vi "CreateChanGrp.vi"(8 "error in (no error)":errorcluster, 9 "GroupChans":refnum<class "Channel.lvclass">[](array[class]), 10 "MeasType":T1, 11 "GroupName":string) -> (0 "error out":errorcluster, 3 "ChanGrp out":refnum<class "ChanGrp.lvclass">)   [LabVIEW 2018, in "Configuration Grandmaster.lvlib" / "ChanGrp.lvclass"]
uses:
  ChanGrp.lvclass
  Custom Ctrls/ge_MeasType.ctl
  Measurements/Class Channel/Channel.lvclass
  ChanGrp.lvclass/ChanGrp.ctl
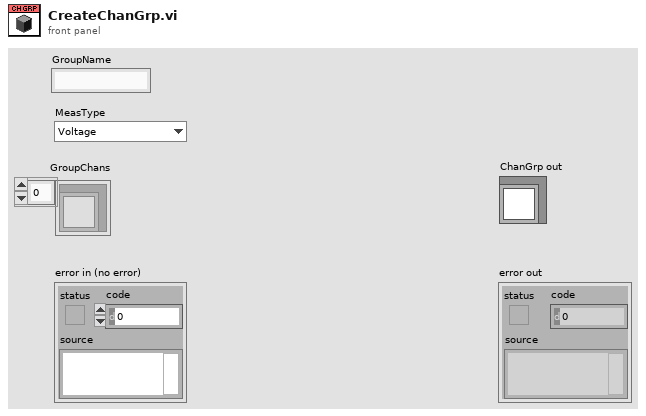
[diagram p1: front panel]
types:
  T1 = typedef "ge_MeasType.ctl" = enum16{"Voltage", "Frequency", "Tachometer", "Dynamic", "Thermocouple", "RTD", "Strain", "Current", "Resistance"}
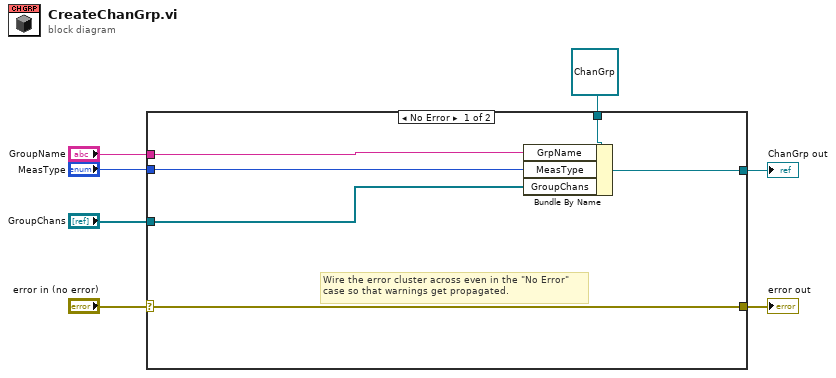
[diagram p0: block diagram]
diagram:
  n1 = case shown="No Error" "error in (no error)" {
    selector: "error in (no error)" -> [w13 w15]
    tunnel: [w13 w15] -> w6
    tunnel: [w11 w14] -> w5
    tunnel: refnum<class "ChanGrp.lvclass"> refnum ("ChanGrp.lvclass") -> [w12 w14]
    tunnel: "GroupName" -> [w10 _]
    tunnel: "MeasType" -> [w9 _]
    tunnel: "GroupChans" -> [w8 _]
    frame No Error {
      # "Wire the error cluster across even in the \"No Error\"\ncase so that warnings get propagated."
      n2 = Bundle By Name(cluster=w12, "GrpName"=w10, "MeasType"=w9, "GroupChans"=w8) -> (w11:refnum<class "ChanGrp.lvclass">)
    }
    frame Error {
    }
  }
  "error out" <- w6
  "ChanGrp out" <- w5
